vi "testcolorsimple.vi"() -> ()   [LabVIEW 2019]
panel:
  out "Classes (Color Classification 1)":string[](array[string])
  in  "Stop (F)":bool
  out "Image Out":T1(plugin-control)
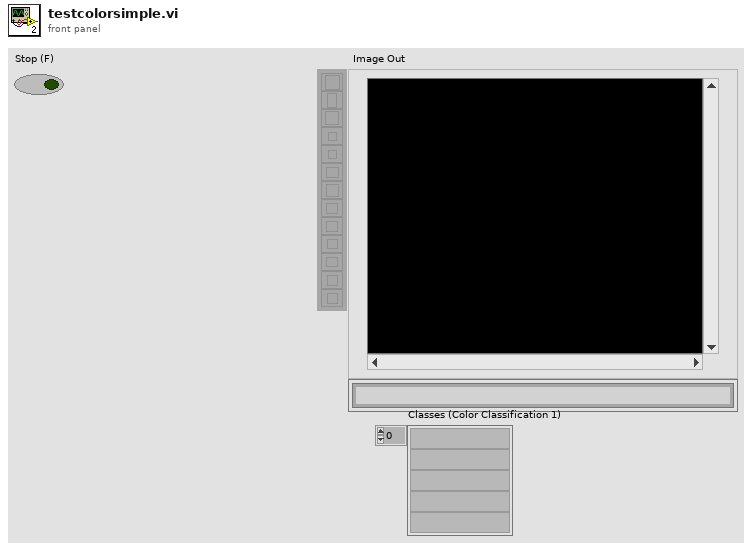
[diagram p1: front panel]
types:
  T1 = typedef "IMAQ Image.ctl" = refnum<image>
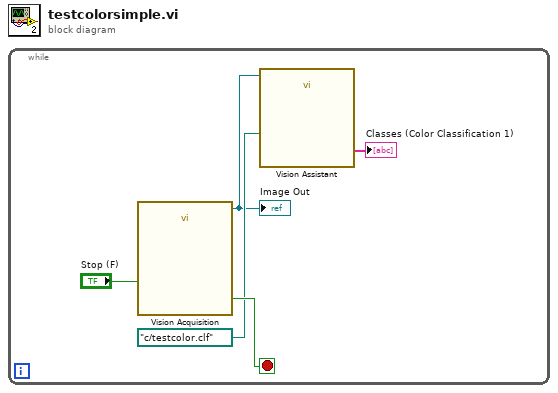
[diagram p0: block diagram]
diagram:
  n1 = while {
    stop <- w4 stop-if-true
    n2 = call "Vision Acquisition"("Stop (F)"="Stop (F)") -> ("Image Out"=w1:T1, "Stopped"=w4:bool)  [unwired: 24 in, 1 out]
    "Image Out" <- w1
    n3 = call "Vision Assistant"("Image In"=w1, "File Path (Color Classification 1)"=path "c:/testcolor.clf") -> ("Classes (Color Classification 1)"=→"Classes (Color Classification 1)":string[])  [unwired: 23 in, 2 out]
  }
